vi "setColor.vi"(0 "reference":refnum<class "NoteNode.lvclass">, 1 "color":u32(colorbox), 5 "error in (no error)":errorcluster) -> (14 "reference out":refnum<class "NoteNode.lvclass">, 19 "error out":errorcluster)   [LabVIEW 2016, in "NoteNode.lvclass"]
doc: "public void setColor(Color newValue)"
uses:
  <resource>/Framework/Providers/Open_GDS/UML/NoteNode_class/NoteNode.lvclass
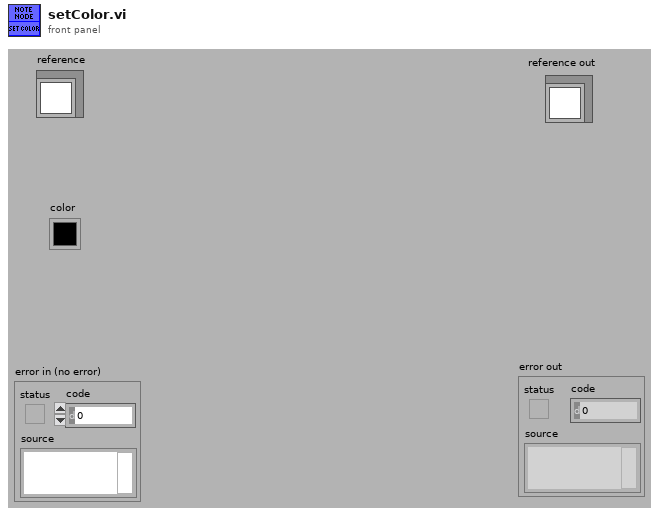
[diagram p1: front panel]
types:
  T1 = typedef "NoteNode.lvclass/ObjectAttributes.ctl" = cluster{"DEFAULT_WIDTH":i32, "DEFAULT_HEIGHT":i32, "DEFAULT_COLOR":u32, "FOLD_X":i32, "FOLD_Y":i32, "color":u32, "text":refnum<class "MultiLineString.lvclass">, "pointNodes":refnum<class "AbstractNode.lvclass">[]}
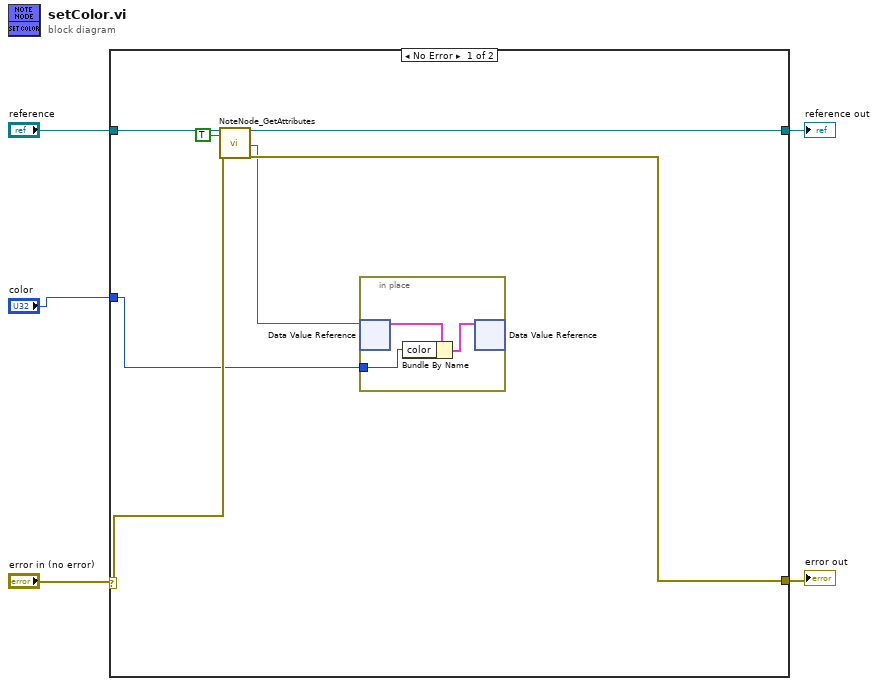
[diagram p0: block diagram]
diagram:
  n1 = case shown="No Error" "error in (no error)" {
    selector: "error in (no error)" -> [w9 w16]
    tunnel: "reference" -> [w12 w17]
    tunnel: [w11 w16] -> w4
    tunnel: [w10 w17] -> w3
    tunnel: "color" -> [w6 _]
    frame No Error {
      n2 = call <resource>:"NoteNode_GetAttributes.vi"("reference in"=w12, "OnlyGetDvrReference(False)"=TRUE, "error in (no error)"=w9) -> ("reference out"=w10:refnum<class "NoteNode.lvclass">, "DataRef"=w7:refnum<data-value>, "error out"=w11:errorcluster)  [unwired: 13 in, 1 out]
      n3 = in-place {
        in-place-border: w6 -> [w14]
        n4 = in-place-dvr #1(w7) -> (w15:T1)  [unwired: 1 out]
        n5 = Bundle By Name(cluster=w15, "color"=w14) -> (w13:T1)
        n6 = in-place-dvr #1(w13) -> ()  [unwired: 2 out]
      }
    }
    frame Error {
    }
  }
  "reference out" <- w3
  "error out" <- w4
